vi "LabVIEW Data to Python String (Variant).vi"(8 "error in (no error)":errorcluster, 10 "LabVIEW Data":variant) -> (0 "error out":errorcluster, 2 "Python String":string)   [LabVIEW 2020, in "jki_python_data_tools.lvlib"]
uses:
  jki_python_data_tools.lvlib
  <userlib>/_OpenG.lib/lvdata/lvdata.llb/openg_variant.lvlib
  <userlib>/_OpenG.lib/string/string.llb/openg_string.lvlib
panel:
  # "Copyright © 2003-2009 JKI. All rights reserved.\n\nAuthor: Jim Kring [jim.kring@jameskring.com]\n\nThis library is provided \"AS IS\" ,WITHOUT WARRANTIES OR \nCONDITIONS OF ANY KIND, either express or implied.\n\nJames Kring, Inc. -- http://www.jameskring.com"
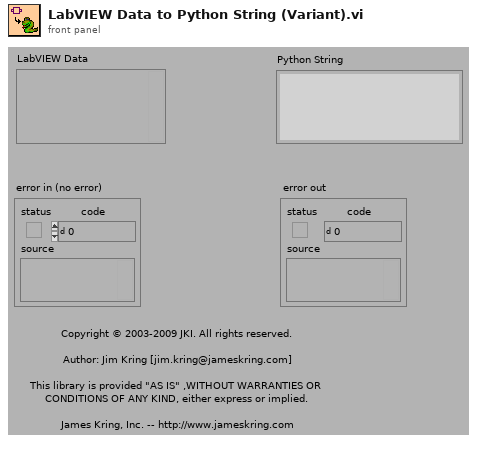
[diagram p1: front panel]
types:
  T1 = typedef "openg_variant.lvlib/Type Descriptor Enumeration__ogtk.ctl" = enum8{"<Null>", "I8", "I16", "I32", "I64", "U8", "U16", "U32", "U64", "SGL", "DBL", "EXT", "CSG", "CDB", "CXT", "0x0F", "0x10", "0x11", "0x12", "0x13", "0x14", "Enum U8", "Enum U16", "Enum U32", "Enum U64", "SGL PQ", "DBL PQ", "EXT PQ", "CSG PQ", "CDB PQ", "CXT PQ", "0x1F", "0x20", "Boolean", "0x22", "0x23", "0x24", "0x25", "0x26", "0x27", "0x28", "0x29", "0x2A", "0x2B", "0x2C", "0x2D", "0x2E", "0x2F", "String", "0x31", "Path", "Pict", "0x34", "0x35", "0x36", "DAQ", "0x38", "0x39", "0x3A", "0x3B", "0x3C", "0x3D", "0x3E", "0x3F", "Array", "0x41", "0x42", "0x43", "0x44", "0x45", "0x46", "0x47", "0x48", "0x49", "0x4A", "0x4B", "0x4C", "0x4D", "0x4E", "0x4F", "Cluster", "0x51", "0x52", "Variant", "Waveform", "0x55", "0x56", "0x57", "0x58", "0x59", "0x5A", "0x5B", "0x5C", "0x5D", "0x5E", "Fixed Point", "0x60", "0x61", "0x62", "0x63", "0x64", "0x65", "0x66", "0x67", "0x68", "0x69", "0x6A", "0x6B", "0x6C", "0x6D", "0x6E", "0x6F", "Refnum", "0x71", "0x72", "Set Collection", "Map Collection"}
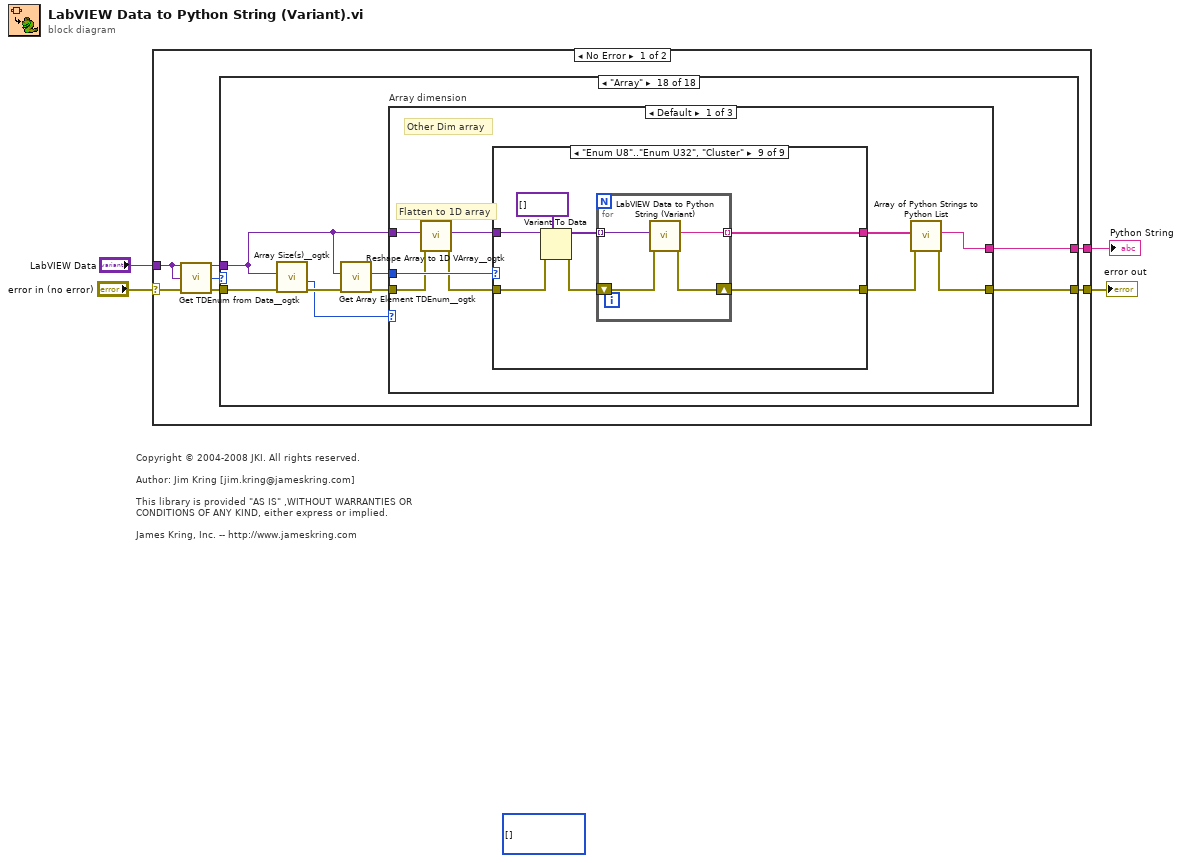
[diagram p0: block diagram]
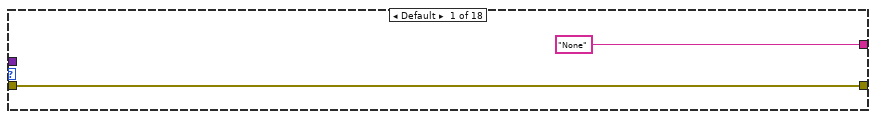
[diagram p2: hidden frame]
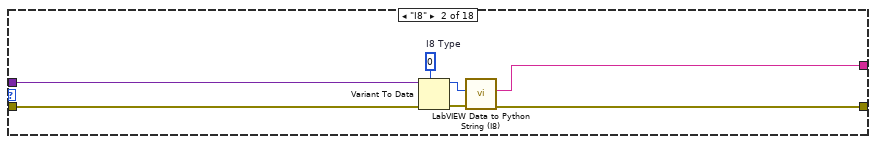
[diagram p3: hidden frame]
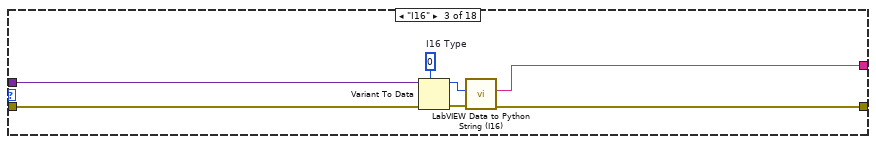
[diagram p4: hidden frame]
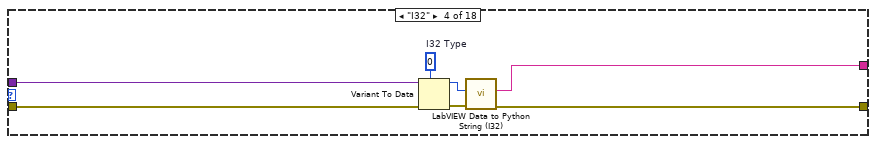
[diagram p5: hidden frame]
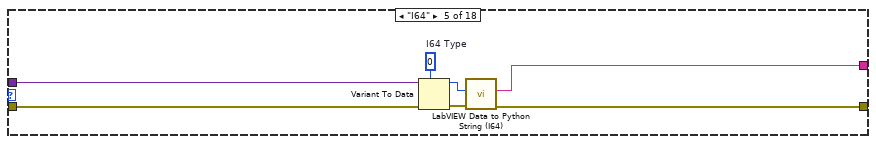
[diagram p6: hidden frame]
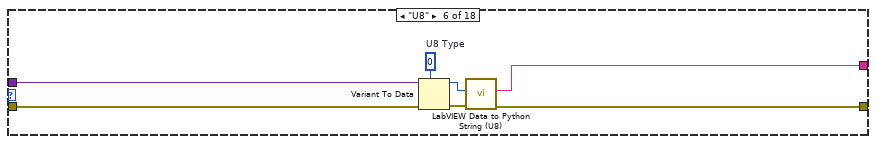
[diagram p7: hidden frame]
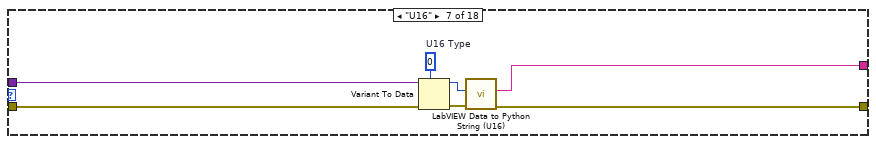
[diagram p8: hidden frame]
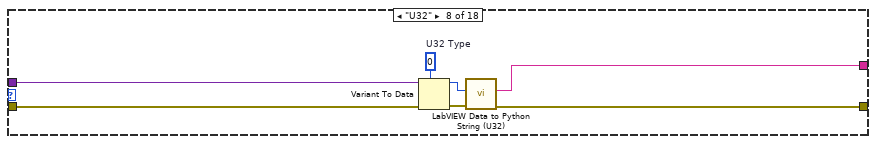
[diagram p9: hidden frame]
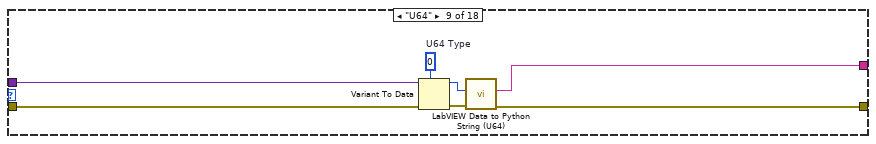
[diagram p10: hidden frame]
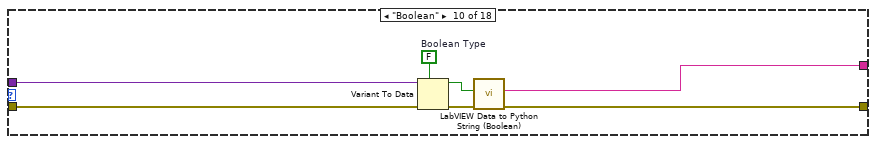
[diagram p11: hidden frame]
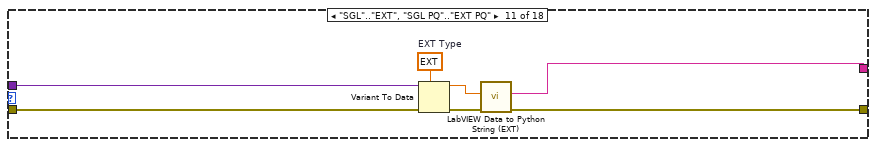
[diagram p12: hidden frame]
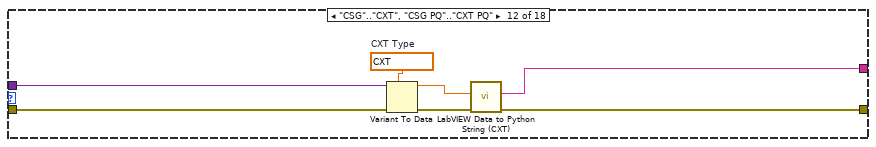
[diagram p13: hidden frame]
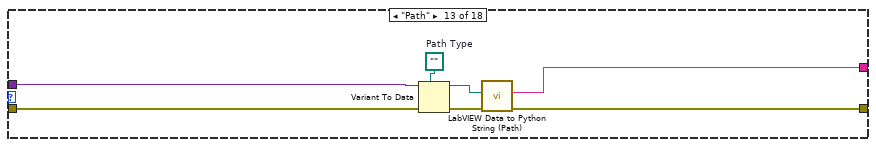
[diagram p14: hidden frame]
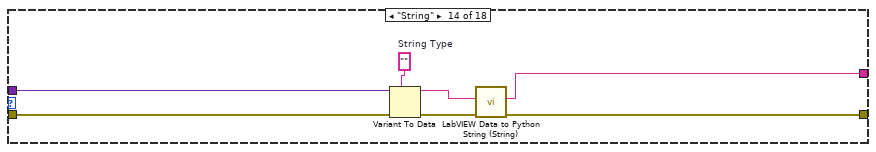
[diagram p15: hidden frame]
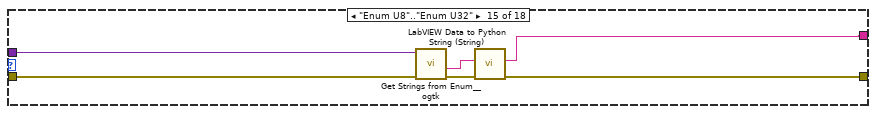
[diagram p16: hidden frame]
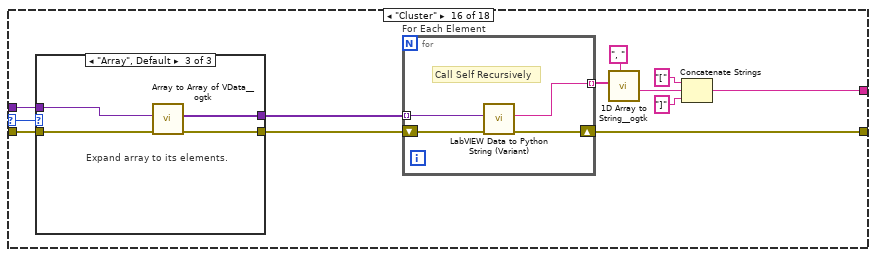
[diagram p17: hidden frame]
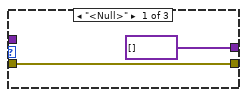
[diagram p18: hidden frame]
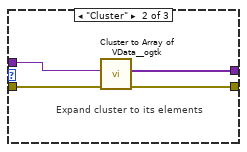
[diagram p19: hidden frame]
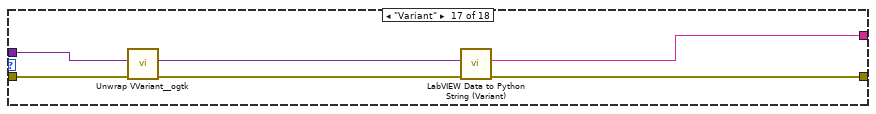
[diagram p20: hidden frame]
diagram:
  (unwired) i32[] []
  # "Copyright © 2004-2008 JKI. All rights reserved.\n\nAuthor: Jim Kring [jim.kring@jameskring.com]\n\nThis library is provided \"AS IS\" ,WITHOUT WARRANTIES OR \nCONDITIONS OF ANY KIND, either express or implied.\n\nJames Kring, Inc. -- http://www.jameskring.com"
  n1 = case shown="No Error" "error in (no error)" {
    selector: "error in (no error)" -> [w8 w547]
    tunnel: [w5 w547] -> w4
    tunnel: "LabVIEW Data" -> [w7 _]
    tunnel: [w6 "None"] -> w1
    frame No Error {
      n2 = call <userlib>:"Get TDEnum from Data__ogtk.vi"("Data"=w7) -> ("Type Descriptor Enumeration"=w9:T1)  [unwired: 4 in]
      n3 = case shown="\"Array\"" w9 {
        selector: w9 -> [_ _ _ _ _ _ _ _ _ _ _ _ _ _ _ w111 _ _]
        tunnel: w7 -> [_ w17 w24 w31 w38 w45 w52 w59 w66 w73 w80 w88 w94 w101 w107 w120 w140 w144]
        tunnel: w8 -> [w10 w16 w23 w30 w37 w44 w51 w58 w65 w72 w79 w87 w93 w100 w108 w119 w139 w145]
        tunnel: ["None" w12 w19 w26 w33 w40 w47 w54 w61 w68 w75 w82 w91 w97 w103 w112 w137 w141] -> w6
        tunnel: [w10 w13 w20 w27 w34 w41 w48 w55 w62 w69 w76 w84 w90 w96 w104 w110 w136 w142] -> w5
        frame Default {
        }
        frame "I8" {
          w18 = i8 0  # I8 Type
          n4 = Variant To Data(error in=w16, type=w18, Variant=w17) -> (data=w15:i8, error out=w14:errorcluster)
          n5 = call "LabVIEW Data to Python String (I8).vi"("error in (no error)"=w14, "LabVIEW Data"=w15) -> ("error out"=w13:errorcluster, "Python String"=w12:string)  [unwired: 8 in]
        }
        frame "I16" {
          w25 = i16 0  # I16 Type
          n6 = Variant To Data(error in=w23, type=w25, Variant=w24) -> (data=w22:i16, error out=w21:errorcluster)
          n7 = call "LabVIEW Data to Python String (I16).vi"("error in (no error)"=w21, "LabVIEW Data"=w22) -> ("error out"=w20:errorcluster, "Python String"=w19:string)  [unwired: 8 in]
        }
        frame "I32" {
          w32 = 0  # I32 Type
          n8 = Variant To Data(error in=w30, type=w32, Variant=w31) -> (data=w29:i32, error out=w28:errorcluster)
          n9 = call "LabVIEW Data to Python String (I32).vi"("error in (no error)"=w28, "LabVIEW Data"=w29) -> ("error out"=w27:errorcluster, "Python String"=w26:string)  [unwired: 8 in]
        }
        frame "I64" {
          w39 = i64 0  # I64 Type
          n10 = Variant To Data(error in=w37, type=w39, Variant=w38) -> (data=w36:i64, error out=w35:errorcluster)
          n11 = call "LabVIEW Data to Python String (I64).vi"("error in (no error)"=w35, "LabVIEW Data"=w36) -> ("error out"=w34:errorcluster, "Python String"=w33:string)  [unwired: 8 in]
        }
        frame "U8" {
          w46 = u8 0  # U8 Type
          n12 = Variant To Data(error in=w44, type=w46, Variant=w45) -> (data=w43:u8, error out=w42:errorcluster)
          n13 = call "LabVIEW Data to Python String (U8).vi"("error in (no error)"=w42, "LabVIEW Data"=w43) -> ("error out"=w41:errorcluster, "Python String"=w40:string)  [unwired: 8 in]
        }
        frame "U16" {
          w53 = u16 0  # U16 Type
          n14 = Variant To Data(error in=w51, type=w53, Variant=w52) -> (data=w50:u16, error out=w49:errorcluster)
          n15 = call "LabVIEW Data to Python String (U16).vi"("error in (no error)"=w49, "LabVIEW Data"=w50) -> ("error out"=w48:errorcluster, "Python String"=w47:string)  [unwired: 8 in]
        }
        frame "U32" {
          w60 = u32 0  # U32 Type
          n16 = Variant To Data(error in=w58, type=w60, Variant=w59) -> (data=w57:u32, error out=w56:errorcluster)
          n17 = call "LabVIEW Data to Python String (U32).vi"("error in (no error)"=w56, "LabVIEW Data"=w57) -> ("error out"=w55:errorcluster, "Python String"=w54:string)  [unwired: 8 in]
        }
        frame "U64" {
          w67 = u64 0  # U64 Type
          n18 = Variant To Data(error in=w65, type=w67, Variant=w66) -> (data=w64:u64, error out=w63:errorcluster)
          n19 = call "LabVIEW Data to Python String (U64).vi"("error in (no error)"=w63, "LabVIEW Data"=w64) -> ("error out"=w62:errorcluster, "Python String"=w61:string)  [unwired: 8 in]
        }
        frame "Boolean" {
          w74 = FALSE  # Boolean Type
          n20 = Variant To Data(error in=w72, type=w74, Variant=w73) -> (data=w71:bool, error out=w70:errorcluster)
          n21 = call "LabVIEW Data to Python String (Boolean).vi"("error in (no error)"=w70, "LabVIEW Data"=w71) -> ("error out"=w69:errorcluster, "Python String"=w68:string)  [unwired: 8 in]
        }
        frame "SGL".."EXT", "SGL PQ".."EXT PQ" {
          w81 = ext 0.0  # EXT Type
          n22 = Variant To Data(error in=w79, type=w81, Variant=w80) -> (data=w78:ext, error out=w77:errorcluster)
          n23 = call "LabVIEW Data to Python String (EXT).vi"("error in (no error)"=w77, "LabVIEW Data"=w78) -> ("error out"=w76:errorcluster, "Python String"=w75:string)  [unwired: 8 in]
        }
        frame "CSG".."CXT", "CSG PQ".."CXT PQ" {
          w85 = cxt 0.0+0.0i  # CXT Type
          n24 = Variant To Data(error in=w87, type=w85, Variant=w88) -> (data=w83:cxt, error out=w86:errorcluster)
          n25 = call "LabVIEW Data to Python String (CXT).vi"("error in (no error)"=w86, "LabVIEW Data"=w83) -> ("error out"=w84:errorcluster, "Python String"=w82:string)  [unwired: 8 in]
        }
        frame "Path" {
          w95 = path ""  # Path Type
          n26 = Variant To Data(error in=w93, type=w95, Variant=w94) -> (data=w89:path, error out=w92:errorcluster)
          n27 = call "LabVIEW Data to Python String (Path).vi"("error in (no error)"=w92, "LabVIEW Data"=w89) -> ("error out"=w90:errorcluster, "Python String"=w91:string)  [unwired: 8 in]
        }
        frame "String" {
          w102 = ""  # String Type
          n28 = Variant To Data(error in=w100, type=w102, Variant=w101) -> (data=w99:string, error out=w98:errorcluster)
          n29 = call "LabVIEW Data to Python String (String).vi"("error in (no error)"=w98, "LabVIEW Data"=w99) -> ("error out"=w96:errorcluster, "Python String"=w97:string)  [unwired: 8 in]
        }
        frame "Enum U8".."Enum U32" {
          n30 = call <userlib>:"Get Strings from Enum__ogtk.vi"("error in (no error)"=w108, "Enum"=w107) -> ("error out"=w105:errorcluster, "String Value"=w106:string)  [unwired: 6 in, 2 out]
          n31 = call "LabVIEW Data to Python String (String).vi"("error in (no error)"=w105, "LabVIEW Data"=w106) -> ("error out"=w104:errorcluster, "Python String"=w103:string)  [unwired: 8 in]
        }
        frame "Cluster" {
          n32 = case shown="\"Array\", Default" w111 {
            tunnel: w120 -> [_ w126 w128]
            tunnel: w119 -> [w121 w125 w127]
            tunnel: [variant[] [] w123 w130] -> w118
            tunnel: [w121 w124 w129] -> w109
            frame "<Null>" {
            }
            frame "Cluster" {
              # "Expand cluster to its elements"
              n33 = call <userlib>:"Cluster to Array of VData__ogtk.vi"("error in (no error)"=w125, "Cluster"=w126) -> ("error out"=w124:errorcluster, "Array of VData"=w123:variant[])  [unwired: 8 in]
            }
            frame "Array", Default {
              # "Expand array to its elements."
              n34 = call <userlib>:"Array to Array of VData__ogtk.vi"("error in (no error)"=w127, "MultiD Array"=w128) -> ("error out"=w129:errorcluster, "1D Array of Variants"=w130:variant[])  [unwired: 8 in]
            }
          }
          n35 = for "For Each Element" {
            shift-right: [w132] -> w110
            shift-left: w109 -> [w131]
            tunnel: w118 -> [w134] mode=indexing
            tunnel: [w133] -> w117 mode=indexing
            # "Call Self Recursively"
            n36 = call "LabVIEW Data to Python String (Variant).vi"("error in (no error)"=w131, "LabVIEW Data"=w134) -> ("error out"=w132:errorcluster, "Python String"=w133:string)  [unwired: 8 in]
          }
          n37 = call <userlib>:"1D Array to String__ogtk.vi"("delimiter (Tab)"=", ", "Array of Strings"=w117) -> ("delimited string"=w115:string)  [unwired: 9 in]
          n38 = Concatenate Strings("[" ("string"), w115, "]" ("string")) -> (w112:string)
        }
        frame "Variant" {
          n39 = call <userlib>:"Unwrap VVariant__ogtk.vi"("error in (no error)"=w139, "VVariant"=w140) -> ("error out"=w135:errorcluster, "Variant"=w138:variant)  [unwired: 8 in]
          n40 = call "LabVIEW Data to Python String (Variant).vi"("error in (no error)"=w135, "LabVIEW Data"=w138) -> ("error out"=w136:errorcluster, "Python String"=w137:string)  [unwired: 8 in]
        }
        frame "Array" {
          n41 = call <userlib>:"Array Size(s)__ogtk.vi"("error in (no error)"=w145, "Array"=w144) -> ("error out"=w146:errorcluster, "N dims"=w143:u32)  [unwired: 7 in, 1 out]
          n42 = call <userlib>:"Get Array Element TDEnum__ogtk.vi"("error in (no error)"=w146, "Array"=w144) -> ("error out"=w148:errorcluster, "Element Type"=w147:T1)  [unwired: 8 in]
          n43 = case "Array dimension" shown="Default" w143 {
            tunnel: w148 -> [w156 w256 w420]
            tunnel: w147 -> [w157 w255 w421]
            tunnel: [w152 w251 w417] -> w141
            tunnel: [w150 w252 w415] -> w142
            tunnel: w144 -> [w154 w254 w419]
            frame Default {
              # "Flatten to 1D array"
              # "Other Dim array"
              n44 = call <userlib>:"Reshape Array to 1D VArray__ogtk.vi"("error in (no error)"=w156, "MultiD Array"=w154) -> ("error out"=w155:errorcluster, "1D VArray"=w153:variant)  [unwired: 7 in, 1 out]
              n45 = case shown="\"Enum U8\"..\"Enum U32\", \"Cluster\"" w157 {
                tunnel: w153 -> [w164 w169 w183 w193 w205 w215 w226 _ w241]
                tunnel: w155 -> [w158 w170 w182 w194 w204 w216 w227 w235 w243]
                tunnel: [w162 w171 w180 w192 w202 w214 w224 w236 w245] -> w151
                tunnel: [w159 w172 w181 w191 w203 w213 w225 w235 w244] -> w149
                frame "I8".."I64" {
                  n46 = Variant To Data(error in=w158, type=i32[] [], Variant=w164) -> (data=w163:i32[], error out=w160:errorcluster)
                  n47 = for {
                    tunnel: w163 -> [w168] mode=indexing
                    tunnel: [w167] -> w162 mode=indexing
                    shift-right: [w165] -> w159
                    shift-left: w160 -> [w166]
                    n48 = call "LabVIEW Data to Python String (I64).vi"("error in (no error)"=w166, "LabVIEW Data"=w168) -> ("error out"=w165:errorcluster, "Python String"=w167:string)  [unwired: 8 in]
                  }
                }
                frame "U8".."U64" {
                  n49 = Variant To Data(error in=w170, type=u32[] [], Variant=w169) -> (data=w175:u32[], error out=w173:errorcluster)
                  n50 = for {
                    tunnel: w175 -> [w179] mode=indexing
                    tunnel: [w178] -> w171 mode=indexing
                    shift-right: [w176] -> w172
                    shift-left: w173 -> [w177]
                    n51 = call "LabVIEW Data to Python String (U64).vi"("error in (no error)"=w177, "LabVIEW Data"=w179) -> ("error out"=w176:errorcluster, "Python String"=w178:string)  [unwired: 8 in]
                  }
                }
                frame "Boolean" {
                  n52 = Variant To Data(error in=w182, type=bool[] [], Variant=w183) -> (data=w186:bool[], error out=w184:errorcluster)
                  n53 = for {
                    tunnel: w186 -> [w190] mode=indexing
                    tunnel: [w189] -> w180 mode=indexing
                    shift-right: [w187] -> w181
                    shift-left: w184 -> [w188]
                    n54 = call "LabVIEW Data to Python String (Boolean).vi"("error in (no error)"=w188, "LabVIEW Data"=w190) -> ("error out"=w187:errorcluster, "Python String"=w189:string)  [unwired: 8 in]
                  }
                }
                frame "SGL".."EXT", "SGL PQ".."EXT PQ" {
                  n55 = Variant To Data(error in=w194, type=ext[] [], Variant=w193) -> (data=w197:ext[], error out=w195:errorcluster)
                  n56 = for {
                    tunnel: w197 -> [w201] mode=indexing
                    tunnel: [w200] -> w192 mode=indexing
                    shift-right: [w198] -> w191
                    shift-left: w195 -> [w199]
                    n57 = call "LabVIEW Data to Python String (EXT).vi"("error in (no error)"=w199, "LabVIEW Data"=w201) -> ("error out"=w198:errorcluster, "Python String"=w200:string)  [unwired: 8 in]
                  }
                }
                frame "CSG".."CXT", "CSG PQ".."CXT PQ" {
                  n58 = Variant To Data(error in=w204, type=cxt[] [], Variant=w205) -> (data=w208:cxt[], error out=w206:errorcluster)
                  n59 = for {
                    tunnel: w208 -> [w212] mode=indexing
                    tunnel: [w211] -> w202 mode=indexing
                    shift-right: [w209] -> w203
                    shift-left: w206 -> [w210]
                    n60 = call "LabVIEW Data to Python String (CXT).vi"("error in (no error)"=w210, "LabVIEW Data"=w212) -> ("error out"=w209:errorcluster, "Python String"=w211:string)  [unwired: 8 in]
                  }
                }
                frame "Path" {
                  n61 = Variant To Data(error in=w216, type=path[] [], Variant=w215) -> (data=w219:path[], error out=w217:errorcluster)
                  n62 = for {
                    tunnel: w219 -> [w223] mode=indexing
                    tunnel: [w222] -> w214 mode=indexing
                    shift-right: [w220] -> w213
                    shift-left: w217 -> [w221]
                    n63 = call "LabVIEW Data to Python String (Path).vi"("error in (no error)"=w221, "LabVIEW Data"=w223) -> ("error out"=w220:errorcluster, "Python String"=w222:string)  [unwired: 8 in]
                  }
                }
                frame "String" {
                  n64 = Variant To Data(error in=w227, type=string[] [], Variant=w226) -> (data=w230:string[], error out=w228:errorcluster)
                  n65 = for {
                    tunnel: w230 -> [w234] mode=indexing
                    tunnel: [w233] -> w224 mode=indexing
                    shift-right: [w231] -> w225
                    shift-left: w228 -> [w232]
                    n66 = call "LabVIEW Data to Python String (String).vi"("error in (no error)"=w232, "LabVIEW Data"=w234) -> ("error out"=w231:errorcluster, "Python String"=w233:string)  [unwired: 8 in]
                  }
                }
                frame Default {
                  n67 = Initialize Array("", 0 ("dimension size")) -> (w236:string[])
                }
                frame "Enum U8".."Enum U32", "Cluster" {
                  n68 = Variant To Data(error in=w243, type=variant[] [] ("1D Array of Variants"), Variant=w241) -> (data=w240:variant[], error out=w242:errorcluster)
                  n69 = for {
                    shift-right: [w247] -> w244
                    shift-left: w242 -> [w248]
                    tunnel: w240 -> [w249] mode=indexing
                    tunnel: [w246] -> w245 mode=indexing
                    n70 = call "LabVIEW Data to Python String (Variant).vi"("error in (no error)"=w248, "LabVIEW Data"=w249) -> ("error out"=w247:errorcluster, "Python String"=w246:string)  [unwired: 8 in]
                  }
                }
              }
              n71 = call "Array of Python Strings to Python List.vi"("error in (no error)"=w149, "Array of Python Strings"=w151) -> ("error out"=w150:errorcluster, "Python List"=w152:string)  [unwired: 8 in]
            }
            frame 1 {
              # "1D array"
              n72 = case shown="\"Enum U8\"..\"Enum U32\", \"Cluster\"" w255 {
                tunnel: w254 -> [w263 w274 w285 w296 w307 w318 w329 w340 w348 w358 w368 w380 w391 _ w406]
                tunnel: w256 -> [w257 w268 w279 w290 w301 w312 w323 w334 w347 w359 w367 w381 w392 w403 w408]
                tunnel: [w261 w272 w283 w294 w305 w316 w327 w338 w345 w357 w369 w379 w390 w400 w410] -> w250
                tunnel: [w258 w269 w280 w291 w302 w313 w324 w335 w346 w356 w370 w378 w389 w403 w409] -> w253
                frame "I8" {
                  n73 = Variant To Data(error in=w257, type=i8[] [], Variant=w263) -> (data=w262:i8[], error out=w259:errorcluster)
                  n74 = for {
                    tunnel: w262 -> [w265] mode=indexing
                    tunnel: [w264] -> w261 mode=indexing
                    shift-right: [w267] -> w258
                    shift-left: w259 -> [w266]
                    n75 = call "LabVIEW Data to Python String (I8).vi"("error in (no error)"=w266, "LabVIEW Data"=w265) -> ("error out"=w267:errorcluster, "Python String"=w264:string)  [unwired: 8 in]
                  }
                }
                frame "I16" {
                  n76 = Variant To Data(error in=w268, type=i16[] [], Variant=w274) -> (data=w273:i16[], error out=w270:errorcluster)
                  n77 = for {
                    tunnel: w273 -> [w276] mode=indexing
                    tunnel: [w275] -> w272 mode=indexing
                    shift-right: [w278] -> w269
                    shift-left: w270 -> [w277]
                    n78 = call "LabVIEW Data to Python String (I16).vi"("error in (no error)"=w277, "LabVIEW Data"=w276) -> ("error out"=w278:errorcluster, "Python String"=w275:string)  [unwired: 8 in]
                  }
                }
                frame "I32" {
                  n79 = Variant To Data(error in=w279, type=i32[] [], Variant=w285) -> (data=w284:i32[], error out=w281:errorcluster)
                  n80 = for {
                    tunnel: w284 -> [w287] mode=indexing
                    tunnel: [w286] -> w283 mode=indexing
                    shift-right: [w289] -> w280
                    shift-left: w281 -> [w288]
                    n81 = call "LabVIEW Data to Python String (I32).vi"("error in (no error)"=w288, "LabVIEW Data"=w287) -> ("error out"=w289:errorcluster, "Python String"=w286:string)  [unwired: 8 in]
                  }
                }
                frame "I64" {
                  n82 = Variant To Data(error in=w290, type=i64[] [], Variant=w296) -> (data=w295:i64[], error out=w292:errorcluster)
                  n83 = for {
                    tunnel: w295 -> [w298] mode=indexing
                    tunnel: [w297] -> w294 mode=indexing
                    shift-right: [w300] -> w291
                    shift-left: w292 -> [w299]
                    n84 = call "LabVIEW Data to Python String (I64).vi"("error in (no error)"=w299, "LabVIEW Data"=w298) -> ("error out"=w300:errorcluster, "Python String"=w297:string)  [unwired: 8 in]
                  }
                }
                frame "U8" {
                  n85 = Variant To Data(error in=w301, type=u8[] [], Variant=w307) -> (data=w306:u8[], error out=w303:errorcluster)
                  n86 = for {
                    tunnel: w306 -> [w309] mode=indexing
                    tunnel: [w308] -> w305 mode=indexing
                    shift-right: [w311] -> w302
                    shift-left: w303 -> [w310]
                    n87 = call "LabVIEW Data to Python String (U8).vi"("error in (no error)"=w310, "LabVIEW Data"=w309) -> ("error out"=w311:errorcluster, "Python String"=w308:string)  [unwired: 8 in]
                  }
                }
                frame "U16" {
                  n88 = Variant To Data(error in=w312, type=u16[] [], Variant=w318) -> (data=w317:u16[], error out=w314:errorcluster)
                  n89 = for {
                    tunnel: w317 -> [w320] mode=indexing
                    tunnel: [w319] -> w316 mode=indexing
                    shift-right: [w322] -> w313
                    shift-left: w314 -> [w321]
                    n90 = call "LabVIEW Data to Python String (U16).vi"("error in (no error)"=w321, "LabVIEW Data"=w320) -> ("error out"=w322:errorcluster, "Python String"=w319:string)  [unwired: 8 in]
                  }
                }
                frame "U32" {
                  n91 = Variant To Data(error in=w323, type=u32[] [], Variant=w329) -> (data=w328:u32[], error out=w325:errorcluster)
                  n92 = for {
                    tunnel: w328 -> [w331] mode=indexing
                    tunnel: [w330] -> w327 mode=indexing
                    shift-right: [w333] -> w324
                    shift-left: w325 -> [w332]
                    n93 = call "LabVIEW Data to Python String (U32).vi"("error in (no error)"=w332, "LabVIEW Data"=w331) -> ("error out"=w333:errorcluster, "Python String"=w330:string)  [unwired: 8 in]
                  }
                }
                frame "U64" {
                  n94 = Variant To Data(error in=w334, type=u64[] [], Variant=w340) -> (data=w339:u64[], error out=w336:errorcluster)
                  n95 = for {
                    tunnel: w339 -> [w342] mode=indexing
                    tunnel: [w341] -> w338 mode=indexing
                    shift-right: [w344] -> w335
                    shift-left: w336 -> [w343]
                    n96 = call "LabVIEW Data to Python String (U64).vi"("error in (no error)"=w343, "LabVIEW Data"=w342) -> ("error out"=w344:errorcluster, "Python String"=w341:string)  [unwired: 8 in]
                  }
                }
                frame "Boolean" {
                  n97 = Variant To Data(error in=w347, type=bool[] [], Variant=w348) -> (data=w351:bool[], error out=w349:errorcluster)
                  n98 = for {
                    tunnel: w351 -> [w355] mode=indexing
                    tunnel: [w354] -> w345 mode=indexing
                    shift-right: [w352] -> w346
                    shift-left: w349 -> [w353]
                    n99 = call "LabVIEW Data to Python String (Boolean).vi"("error in (no error)"=w353, "LabVIEW Data"=w355) -> ("error out"=w352:errorcluster, "Python String"=w354:string)  [unwired: 8 in]
                  }
                }
                frame "SGL".."EXT", "SGL PQ".."EXT PQ" {
                  n100 = Variant To Data(error in=w359, type=ext[] [], Variant=w358) -> (data=w362:ext[], error out=w360:errorcluster)
                  n101 = for {
                    tunnel: w362 -> [w366] mode=indexing
                    tunnel: [w365] -> w357 mode=indexing
                    shift-right: [w363] -> w356
                    shift-left: w360 -> [w364]
                    n102 = call "LabVIEW Data to Python String (EXT).vi"("error in (no error)"=w364, "LabVIEW Data"=w366) -> ("error out"=w363:errorcluster, "Python String"=w365:string)  [unwired: 8 in]
                  }
                }
                frame "CSG".."CXT", "CSG PQ".."CXT PQ" {
                  n103 = Variant To Data(error in=w367, type=cxt[] [], Variant=w368) -> (data=w373:cxt[], error out=w371:errorcluster)
                  n104 = for {
                    tunnel: w373 -> [w377] mode=indexing
                    tunnel: [w376] -> w369 mode=indexing
                    shift-right: [w374] -> w370
                    shift-left: w371 -> [w375]
                    n105 = call "LabVIEW Data to Python String (CXT).vi"("error in (no error)"=w375, "LabVIEW Data"=w377) -> ("error out"=w374:errorcluster, "Python String"=w376:string)  [unwired: 8 in]
                  }
                }
                frame "Path" {
                  n106 = Variant To Data(error in=w381, type=path[] [], Variant=w380) -> (data=w384:path[], error out=w382:errorcluster)
                  n107 = for {
                    tunnel: w384 -> [w388] mode=indexing
                    tunnel: [w387] -> w379 mode=indexing
                    shift-right: [w385] -> w378
                    shift-left: w382 -> [w386]
                    n108 = call "LabVIEW Data to Python String (Path).vi"("error in (no error)"=w386, "LabVIEW Data"=w388) -> ("error out"=w385:errorcluster, "Python String"=w387:string)  [unwired: 8 in]
                  }
                }
                frame "String" {
                  n109 = Variant To Data(error in=w392, type=string[] [], Variant=w391) -> (data=w395:string[], error out=w393:errorcluster)
                  n110 = for {
                    tunnel: w395 -> [w399] mode=indexing
                    tunnel: [w398] -> w390 mode=indexing
                    shift-right: [w396] -> w389
                    shift-left: w393 -> [w397]
                    n111 = call "LabVIEW Data to Python String (String).vi"("error in (no error)"=w397, "LabVIEW Data"=w399) -> ("error out"=w396:errorcluster, "Python String"=w398:string)  [unwired: 8 in]
                  }
                }
                frame Default {
                  n112 = Initialize Array("", 0 ("dimension size")) -> (w400:string[])
                }
                frame "Enum U8".."Enum U32", "Cluster" {
                  n113 = Variant To Data(error in=w408, type=variant[] [] ("1D Array of Variants"), Variant=w406) -> (data=w405:variant[], error out=w407:errorcluster)
                  n114 = for {
                    shift-right: [w412] -> w409
                    shift-left: w407 -> [w413]
                    tunnel: w405 -> [w414] mode=indexing
                    tunnel: [w411] -> w410 mode=indexing
                    n115 = call "LabVIEW Data to Python String (Variant).vi"("error in (no error)"=w413, "LabVIEW Data"=w414) -> ("error out"=w412:errorcluster, "Python String"=w411:string)  [unwired: 8 in]
                  }
                }
              }
              n116 = call "Array of Python Strings to Python List.vi"("error in (no error)"=w253, "Array of Python Strings"=w250) -> ("error out"=w252:errorcluster, "Python List"=w251:string)  [unwired: 8 in]
            }
            frame 2 {
              # "2D array"
              n117 = case shown="\"Enum U8\"..\"Enum U32\", \"Cluster\"" w421 {
                tunnel: w419 -> [w428 w437 w455 w469 w483 w499 w514 _ w533]
                tunnel: w420 -> [w422 w438 w454 w470 w482 w500 w515 w530 w535]
                tunnel: [w426 w439 w452 w468 w484 w498 w513 w528 w537] -> w418
                tunnel: [w423 w440 w453 w467 w485 w497 w512 w530 w536] -> w416
                frame "I8".."I64" {
                  n118 = Variant To Data(error in=w422, type=i32[][] [], Variant=w428) -> (data=w427:i32[][], error out=w424:errorcluster)
                  n119 = for {
                    tunnel: w427 -> [w432] mode=indexing
                    tunnel: [w429] -> w426 mode=indexing
                    shift-right: [w430] -> w423
                    shift-left: w424 -> [w431]
                    n120 = for {
                      tunnel: w432 -> [w436] mode=indexing
                      tunnel: [w435] -> w429 mode=indexing
                      shift-right: [w433] -> w430
                      shift-left: w431 -> [w434]
                      n121 = call "LabVIEW Data to Python String (I64).vi"("error in (no error)"=w434, "LabVIEW Data"=w436) -> ("error out"=w433:errorcluster, "Python String"=w435:string)  [unwired: 8 in]
                    }
                  }
                }
                frame "U8".."U64" {
                  n122 = Variant To Data(error in=w438, type=u32[][] [], Variant=w437) -> (data=w443:u32[][], error out=w441:errorcluster)
                  n123 = for {
                    tunnel: w443 -> [w447] mode=indexing
                    tunnel: [w444] -> w439 mode=indexing
                    shift-right: [w445] -> w440
                    shift-left: w441 -> [w446]
                    n124 = for {
                      tunnel: w447 -> [w451] mode=indexing
                      tunnel: [w450] -> w444 mode=indexing
                      shift-right: [w448] -> w445
                      shift-left: w446 -> [w449]
                      n125 = call "LabVIEW Data to Python String (U64).vi"("error in (no error)"=w449, "LabVIEW Data"=w451) -> ("error out"=w448:errorcluster, "Python String"=w450:string)  [unwired: 8 in]
                    }
                  }
                }
                frame "Boolean" {
                  n126 = Variant To Data(error in=w454, type=bool[][] [], Variant=w455) -> (data=w458:bool[][], error out=w456:errorcluster)
                  n127 = for {
                    tunnel: w458 -> [w462] mode=indexing
                    tunnel: [w459] -> w452 mode=indexing
                    shift-right: [w460] -> w453
                    shift-left: w456 -> [w461]
                    n128 = for {
                      tunnel: w462 -> [w466] mode=indexing
                      tunnel: [w465] -> w459 mode=indexing
                      shift-right: [w463] -> w460
                      shift-left: w461 -> [w464]
                      n129 = call "LabVIEW Data to Python String (Boolean).vi"("error in (no error)"=w464, "LabVIEW Data"=w466) -> ("error out"=w463:errorcluster, "Python String"=w465:string)  [unwired: 8 in]
                    }
                  }
                }
                frame "SGL".."EXT", "SGL PQ".."EXT PQ" {
                  n130 = Variant To Data(error in=w470, type=ext[][] [], Variant=w469) -> (data=w473:ext[][], error out=w471:errorcluster)
                  n131 = for {
                    tunnel: w473 -> [w477] mode=indexing
                    tunnel: [w475] -> w468 mode=indexing
                    shift-right: [w474] -> w467
                    shift-left: w471 -> [w476]
                    n132 = for {
                      tunnel: w477 -> [w481] mode=indexing
                      tunnel: [w480] -> w475 mode=indexing
                      shift-right: [w478] -> w474
                      shift-left: w476 -> [w479]
                      n133 = call "LabVIEW Data to Python String (EXT).vi"("error in (no error)"=w479, "LabVIEW Data"=w481) -> ("error out"=w478:errorcluster, "Python String"=w480:string)  [unwired: 8 in]
                    }
                  }
                }
                frame "CSG".."CXT", "CSG PQ".."CXT PQ" {
                  n134 = Variant To Data(error in=w482, type=cxt[][] [], Variant=w483) -> (data=w488:cxt[][], error out=w486:errorcluster)
                  n135 = for {
                    tunnel: w488 -> [w492] mode=indexing
                    tunnel: [w489] -> w484 mode=indexing
                    shift-right: [w490] -> w485
                    shift-left: w486 -> [w491]
                    n136 = for {
                      tunnel: w492 -> [w496] mode=indexing
                      tunnel: [w495] -> w489 mode=indexing
                      shift-right: [w493] -> w490
                      shift-left: w491 -> [w494]
                      n137 = call "LabVIEW Data to Python String (CXT).vi"("error in (no error)"=w494, "LabVIEW Data"=w496) -> ("error out"=w493:errorcluster, "Python String"=w495:string)  [unwired: 8 in]
                    }
                  }
                }
                frame "Path" {
                  n138 = Variant To Data(error in=w500, type=path[][] [], Variant=w499) -> (data=w503:path[][], error out=w501:errorcluster)
                  n139 = for {
                    tunnel: w503 -> [w507] mode=indexing
                    tunnel: [w504] -> w498 mode=indexing
                    shift-right: [w505] -> w497
                    shift-left: w501 -> [w506]
                    n140 = for {
                      tunnel: w507 -> [w511] mode=indexing
                      tunnel: [w510] -> w504 mode=indexing
                      shift-right: [w508] -> w505
                      shift-left: w506 -> [w509]
                      n141 = call "LabVIEW Data to Python String (Path).vi"("error in (no error)"=w509, "LabVIEW Data"=w511) -> ("error out"=w508:errorcluster, "Python String"=w510:string)  [unwired: 8 in]
                    }
                  }
                }
                frame "String" {
                  n142 = Variant To Data(error in=w515, type=string[][] [], Variant=w514) -> (data=w518:string[][], error out=w516:errorcluster)
                  n143 = for {
                    tunnel: w518 -> [w522] mode=indexing
                    tunnel: [w519] -> w513 mode=indexing
                    shift-right: [w520] -> w512
                    shift-left: w516 -> [w521]
                    n144 = for {
                      tunnel: w522 -> [w526] mode=indexing
                      tunnel: [w525] -> w519 mode=indexing
                      shift-right: [w523] -> w520
                      shift-left: w521 -> [w524]
                      n145 = call "LabVIEW Data to Python String (String).vi"("error in (no error)"=w524, "LabVIEW Data"=w526) -> ("error out"=w523:errorcluster, "Python String"=w525:string)  [unwired: 8 in]
                    }
                  }
                }
                frame Default {
                  w527 = 0 ("dimension size")
                  n146 = Initialize Array("", w527, w527) -> (w528:string[][])
                }
                frame "Enum U8".."Enum U32", "Cluster" {
                  n147 = Variant To Data(error in=w535, type=variant[][] [] ("1D Array of Variants"), Variant=w533) -> (data=w532:variant[][], error out=w534:errorcluster)
                  n148 = for {
                    tunnel: [w538] -> w537 mode=indexing
                    tunnel: w532 -> [w539] mode=indexing
                    shift-right: [w541] -> w536
                    shift-left: w534 -> [w540]
                    n149 = for {
                      shift-right: [w543] -> w541
                      shift-left: w540 -> [w544]
                      tunnel: w539 -> [w545] mode=indexing
                      tunnel: [w542] -> w538 mode=indexing
                      n150 = call "LabVIEW Data to Python String (Variant).vi"("error in (no error)"=w544, "LabVIEW Data"=w545) -> ("error out"=w543:errorcluster, "Python String"=w542:string)  [unwired: 8 in]
                    }
                  }
                }
              }
              n151 = call "2D Array of Python Strings to Python List.vi"("error in (no error)"=w416, "Array of Python Strings"=w418) -> ("error out"=w415:errorcluster, "Python List"=w417:string)  [unwired: 8 in]
            }
          }
        }
      }
    }
    frame Error {
    }
  }
  "error out" <- w4
  "Python String" <- w1
